vi "threshold2gray.vi"(11 "threshold image":T1) -> (3 "grayscale image":T1)   [LabVIEW 2017]
uses:
  <vilib>/vision/Image Controls.llb/IMAQ Image.ctl
  <vilib>/vision/NI_Vision_Development_Module.lvlib
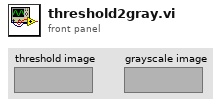
[diagram p1: front panel]
types:
  T1 = typedef "IMAQ Image.ctl" = refnum<image>
  T2 = cluster{"histogram":u32[], "Minimal Value":sgl, "Maximal Value":sgl, "Starting Value":sgl, "Interval Width":sgl, "Mean Value":sgl, "Standard  Variation":sgl, "Area (pixels)":i32}
  T3 = typedef "Image Unit" = enum32{"Undefined", "Angström", "Micrometer", "Millimeter", "Centimeter", "Meter", "Kilometer", "Microinch", "Inch", "Feet", "Nautical miles", "Standard miles", "Steps"}
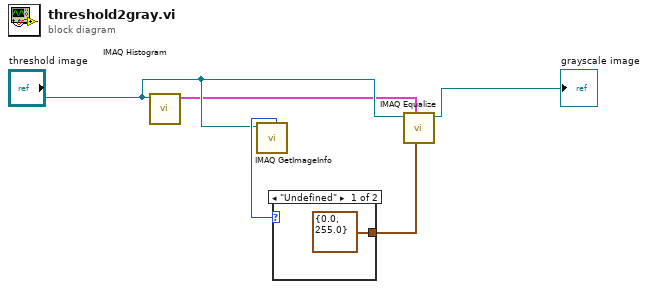
[diagram p0: block diagram]
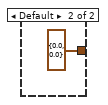
[diagram p2: hidden frame]
diagram:
  n1 = call "IMAQ Histogram"("Image"="threshold image") -> ("Histogram Report"=w2:T2)  [unwired: 4 in, 6 out]
  n2 = call "IMAQ GetImageInfo"("Image"="threshold image") -> ("Unit"=w5:T3)  [unwired: 1 in, 9 out]
  n3 = case shown="\"Undefined\"" w5 {
    tunnel: [cluster{"Minimum":sgl, "Maximum":sgl} {"Minimum"=0.0, "Maximum"=255.0} ("Range") cluster{"Minimum":sgl, "Maximum":sgl} {"Minimum"=0.0, "Maximum"=0.0} ("Range")] -> w1
    frame "Undefined" {
    }
    frame Default {
    }
  }
  n4 = call "IMAQ Equalize"("Range"=w1, "Histogram Report"=w2, "Image Src"="threshold image") -> ("Image Dst Out"=→"grayscale image":T1)  [unwired: 3 in, 5 out]
